vi "ASIC_Configurar valor a 1 canal sumador.vi"(0 "ftHandle_in":u32, 1 "Espera acceso USB":u32=10, 5 "Canal (0..6)":u8 max=6 step=1, 7 "Sumador (0..2)":u8 max=2 step=1, 9 "Valor (OFF-ON)":bool=TRUE, 11 "error in":errorcluster) -> (4 "ftHandle_out":u32, 15 "error out":errorcluster)   [LabVIEW 2009]
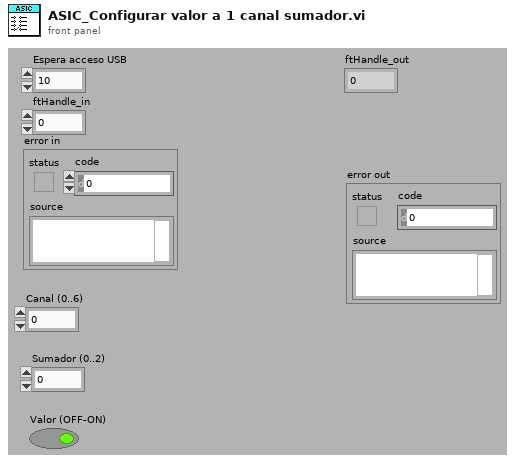
[diagram p1: front panel]
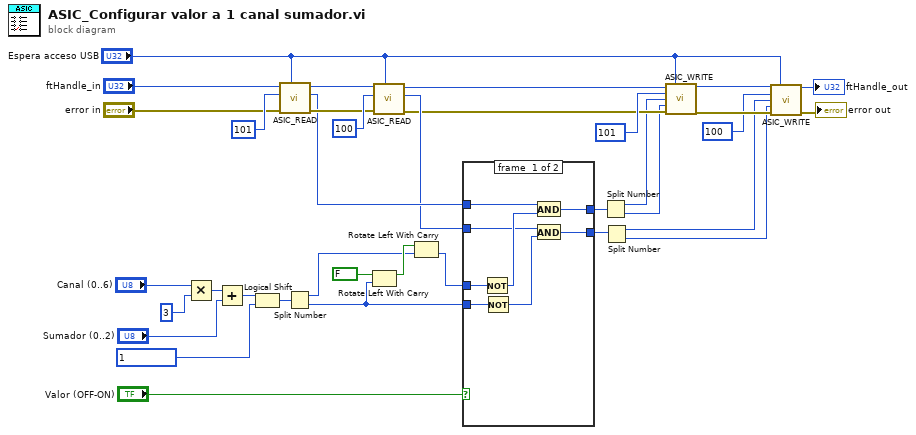
[diagram p0: block diagram]
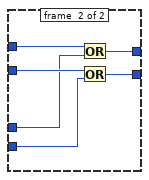
[diagram p2: hidden frame]
diagram:
  n1 = Multiply(x="Canal (0..6)", y=u8 3 ("x")) -> (x*y=w21:u8)
  n2 = Add(x=w21, y="Sumador (0..2)") -> (x+y=w20:u8)
  n3 = Logical Shift(y=w20, x=u32 1 ("x << y")) -> (x << y=w18:u32)
  n4 = call "ASIC_READ.vi"("Espera acceso USB"="Espera acceso USB", "error in"="error in", "Direccion Registro Asic"=u8 101, "ftHandle_in"="ftHandle_in") -> ("error out"=w25:errorcluster, "Valor Asic"=w11:u16, "ftHandle_out"=w29:u32)  [unwired: 5 in]
  n5 = Split Number(x=w18) -> (hi(x)=w15:u16, lo(x)=w13:u16)
  n6 = Rotate Left With Carry(2:w13, 3:FALSE ("carry")) -> (1:w16:bool)  [unwired: 1 out]
  n7 = call "ASIC_READ.vi"("Espera acceso USB"="Espera acceso USB", "error in"=w25, "Direccion Registro Asic"=u8 100, "ftHandle_in"=w29) -> ("error out"=w8:errorcluster, "Valor Asic"=w10:u16, "ftHandle_out"=w9:u32)  [unwired: 5 in]
  n8 = Rotate Left With Carry(2:w15, 3:w16) -> (0:w12:u16)  [unwired: 1 out]
  n9 = case shown="False" "Valor (OFF-ON)" {
    tunnel: w13 -> [w44 w45]
    tunnel: w12 -> [w43 w46]
    tunnel: w11 -> [w42 w50]
    tunnel: w10 -> [w40 w49]
    tunnel: [w38 w48] -> w6
    tunnel: [w37 w47] -> w5
    frame #0 {
      n10 = Not(x=w43) -> (.not. x?=w41:u16)
      n11 = Not(x=w44) -> (.not. x?=w39:u16)
      n12 = And(x=w42, y=w41) -> (x .and. y?=w38:u16)
      n13 = And(x=w40, y=w39) -> (x .and. y?=w37:u16)
    }
    frame #1 {
      n14 = Or(x=w50, y=w46) -> (x .or. y?=w48:u16)
      n15 = Or(x=w49, y=w45) -> (x .or. y?=w47:u16)
    }
  }
  n16 = Split Number(x=w6) -> (hi(x)=w4:u8, lo(x)=w3:u8)
  n17 = Split Number(x=w5) -> (hi(x)=w2:u8, lo(x)=w1:u8)
  n18 = call "ASIC_WRITE.vi"("ftHandle_in"=w9, "Espera acceso USB"="Espera acceso USB", "Direccion Registro Asic"=u8 101, "Byte Alto"=w4, "Byte Bajo"=w3, "error in"=w8) -> ("ftHandle_out"=w36:u32, "error out"=w35:errorcluster)  [unwired: 8 in]
  n19 = call "ASIC_WRITE.vi"("ftHandle_in"=w36, "Espera acceso USB"="Espera acceso USB", "Direccion Registro Asic"=u8 100, "Byte Alto"=w2, "Byte Bajo"=w1, "error in"=w35) -> ("ftHandle_out"=→"ftHandle_out":u32, "error out"=→"error out":errorcluster)  [unwired: 8 in]
